vi "Parse Results Array (all).vi"(6 "Type":T1, 7 "Processing":enum16{"Mean", "Sample"}(ring)=enum."Sample", 8 "error in (no error)":errorcluster, 11 "Results (Dictionary)":cluster{"key":string, "value":dbl[]}[](array[cluster])) -> (0 "error out":errorcluster, 1 "Label":string[](array[string]), 2 "Data":dbl[](array[numeric]), 3 "Results (Dictionary)":cluster{"key":string, "value":dbl[]}[](array[cluster]))   [LabVIEW 2019, in "Instrument.Lockin.lvlib" / "Instrument.Lockin.lvclass"]
doc: "This method will search the <b>Results Dictionary</b> for the data specified by <b>Datatype</b> (X, Y, R, Theta, mean).\n\n<b>Data</b> is an array of clusters, of which each element is an array of the matched datatype."
uses:
  Instrument.Lockin.lvclass
  <vilib>/Analysis/NI_AALBase.lvlib
  <vilib>/Analysis/baseanly.llb/Mean (DBL).vi
  Typedefs/Results Type--Enum.ctl
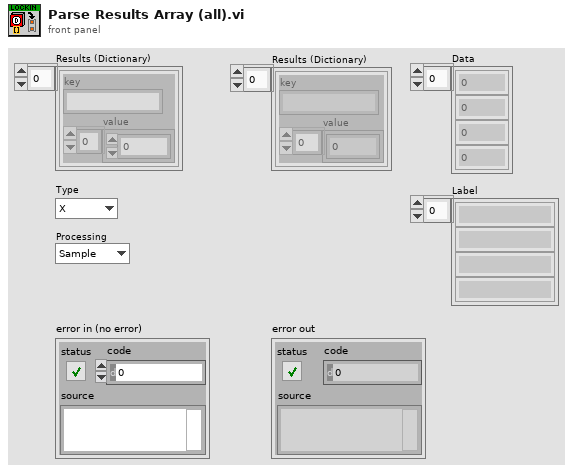
[diagram p1: front panel]
types:
  T1 = typedef "Instrument.Lockin.lvlib/Instrument.Lockin.lvclass/Results Type--Enum.ctl" = enum16{"X", "Y", "R", "Theta", "Mean"}
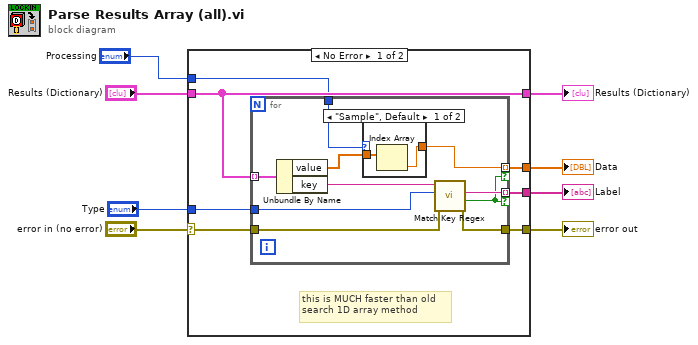
[diagram p0: block diagram]
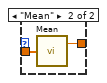
[diagram p2: hidden frame]
diagram:
  n1 = case shown="No Error" "error in (no error)" {
    selector: "error in (no error)" -> [w13 w30]
    tunnel: "Type" -> [w14 _]
    tunnel: "Results (Dictionary)" -> [w15 w31]
    tunnel: [w12 _] -> w6
    tunnel: [w11 w30] -> w3
    tunnel: [w15 w31] -> w5
    tunnel: "Processing" -> [w10 _]
    tunnel: [w9 _] -> w1
    frame No Error {
      # "this is MUCH faster than old\nsearch 1D array method"
      n2 = for {
        tunnel: [w16] -> w9 mode=indexing if=w22
        tunnel: w15 -> [w25] mode=indexing
        tunnel: w14 -> [w19]
        tunnel: w13 -> [w21]
        tunnel: [w23] -> w12 mode=indexing if=w22
        tunnel: [w20] -> w11
        tunnel: w10 -> [w18]
        n3 = Unbundle By Name(w25) -> ("value"=w17:dbl[], "key"=w24:string)
        n4 = case shown="\"Sample\", Default" w18 {
          tunnel: [w27 w29] -> w16
          tunnel: w17 -> [w26 w28]
          frame "Sample", Default {
            n5 = Index Array(array=w26) -> (element=w27:dbl)  [unwired: 1 in]
          }
          frame "Mean" {
            n6 = call-poly <vilib>:"Mean.vi"("X"=w28) -> ("mean"=w29:dbl)  [unwired: 1 out]
          }
        }
        n7 = call "Match Key Regex.vi"("error in"=w21, "Datatype"=w19, "key in"=w24) -> ("error out"=w20:errorcluster, "Datatype Found?"=w22:bool, "Label out"=w23:string)  [unwired: 5 in, 1 out]
      }
    }
    frame Error {
    }
  }
  "Data" <- w1
  "Results (Dictionary)" <- w5
  "Label" <- w6
  "error out" <- w3
